vi "8XY0.vi"(11 "Variables and Memory in":T1 {"GFX" format="%02x"}) -> (3 "Variables and Memory out":T1 {"GFX" format="%02x"})   [LabVIEW 2021]
uses:
  Controls/ClusterF.ctl
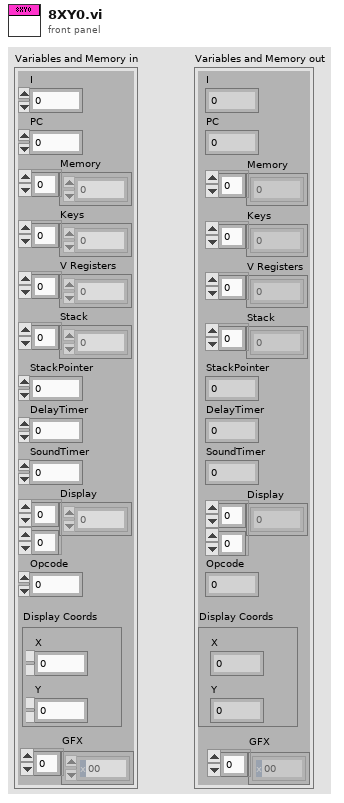
[diagram p1: front panel]
types:
  T1 = typedef "ClusterF.ctl" = cluster{"I":u16, "PC":u16, "Memory":u8[], "Keys":u8[], "V Registers":u8[], "Stack":u16[], "StackPointer":u16, "DelayTimer":u8, "SoundTimer":u8, "Display":u8[][], "Opcode":u16, "Display Coords":cluster{"X":u8, "Y":u8}, "GFX":u8[]}
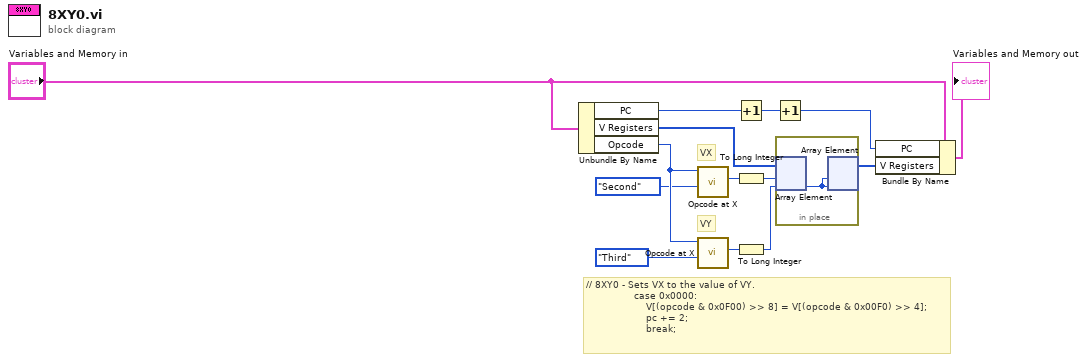
[diagram p0: block diagram]
diagram:
  # "// 8XY0 - Sets VX to the value of VY.\n                case 0x0000:\n                    V[(opcode & 0x0F00) >> 8] = V[(opcode & 0x00F0) >> 4];\n                    pc += 2;\n                    break;"
  # "VX"
  # "VY"
  n1 = Unbundle By Name("Variables and Memory in") -> ("PC"=w9:u16, "V Registers"=w3:u8[], "Opcode"=w14:u16)
  n2 = call "Opcode at X.vi"("X Position"=enum16{"First", "Second", "Third", "Fourth"}."Second", "Opcode"=w14) -> ("Opcode at X Position (U8)"=w4:u8)  [unwired: 9 in]
  n3 = call "Opcode at X.vi"("X Position"=enum16{"First", "Second", "Third", "Fourth"}."Third", "Opcode"=w14) -> ("Opcode at X Position (U8)"=w5:u8)  [unwired: 9 in]
  n4 = Increment(x=w9) -> (x+1=w8:u16)
  n5 = To Long Integer(number=w4) -> (32bit integer=w13:i32)
  n6 = To Long Integer(number=w5) -> (32bit integer=w12:i32)
  n7 = Increment(x=w8) -> (x+1=w10:u16)
  n8 = in-place {
    n9 = in-place-array #1(w3, w13, w12) -> (w15:u8)  [unwired: 1 out]
    n10 = in-place-array #1(w15, w15) -> (w11:u8[])  [unwired: 2 out]
  }
  n11 = Bundle By Name(cluster="Variables and Memory in", "PC"=w10, "V Registers"=w11) -> (→"Variables and Memory out":T1)
